vi "初始化表格.vi"(0 "引用":refnum<vi>) -> ()   [LabVIEW 2015]
uses:
  <vilib>/Utility/miscctls.llb/LVRowAndColumnUnsignedTypeDef.ctl
  <vilib>/Utility/miscctls.llb/LVRowAndColumnTypeDef.ctl
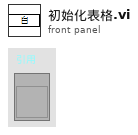
[diagram p1: front panel]
types:
  T1 = typedef "LVRowAndColumnUnsignedTypeDef.ctl" = cluster{"Row":u32, "Column":u32}
  T2 = typedef "LVRowAndColumnTypeDef.ctl" = cluster{"Row":i32, "Column":i32}
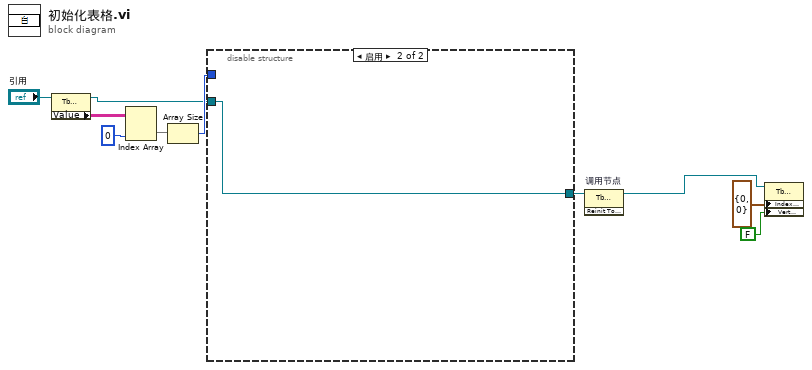
[diagram p0: block diagram]
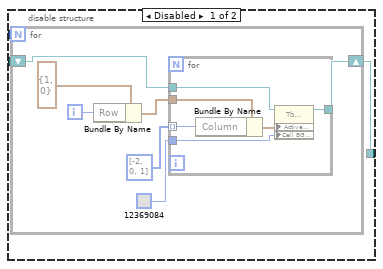
[diagram p2: hidden frame]
diagram:
  n1 = property class="Tbl (严格)"(reference="引用") -> (reference out=w1:refnum<vi>, "Value"=w7:string[][])  [unwired: 1 in, 1 out]
  n2 = Index Array(array=w7, index (col)=0 ("禁用的索引 (列)")) -> (element=w9:string[])  [unwired: 1 in]
  n3 = Array Size(array=w9) -> (size(s)=w10:i32)
  n4 = disable-structure shown="启用" {
    disable-tunnel: w10 -> [w13 _]
    disable-tunnel: [w12 w27] -> w2
    disable-tunnel: w1 -> [w11 w27]
    frame Disabled {
      n5 = for {
        N: w13 -> [_]
        shift-right: [w15] -> w12
        shift-left: w11 -> [w14]
        i -> [w17]
        n6 = Bundle By Name(cluster=T2 {"Row"=1, "Column"=0} ("活动单元格:活动单元格"), "Row"=w17) -> (w18:T2)
        n7 = for {
          tunnel: i32[] [-2, 0, 1] -> [w24] mode=indexing
          tunnel: w18 -> [w25]
          tunnel: u32 12369084 -> [w23]
          tunnel: [w22] -> w15
          tunnel: w14 -> [w21]
          n8 = Bundle By Name(cluster=w25, "Column"=w24) -> (w26:T2)
          n9 = property class="Tbl (严格)"(reference=w21, "Active Cell"=w26, "Cell BG Color"=w23) -> (reference out=w22:refnum<vi>)  [unwired: 1 in, 1 out]
        }
      }
    }
    frame Enabled {
    }
  }
  n10 = invoke on="调用节点" class="Tbl (严格)" method="Reinit To Default"(reference=w2) -> (reference out=w4:refnum<vi>)  [unwired: 2 in, 2 out]
  n11 = property class="Tbl (严格)"(reference=w4, "Index Values"=T1 {"Row"=0, "Column"=0} ("索引值"), "Vert Scrollbar"=FALSE ("显示项:显示垂直滚动条")) -> ()  [unwired: 1 in, 2 out]
